vi "Moving_Avg_Filter.vi"(6 "Moving Array":dbl[][](array[numeric])) -> (3 "Output":dbl, 7 "Coefficients":dbl[](array[numeric]))   [LabVIEW 2016]
panel:
  out "size(s)":i32[](array[numeric])
  in  "Input":dbl[](array[numeric])
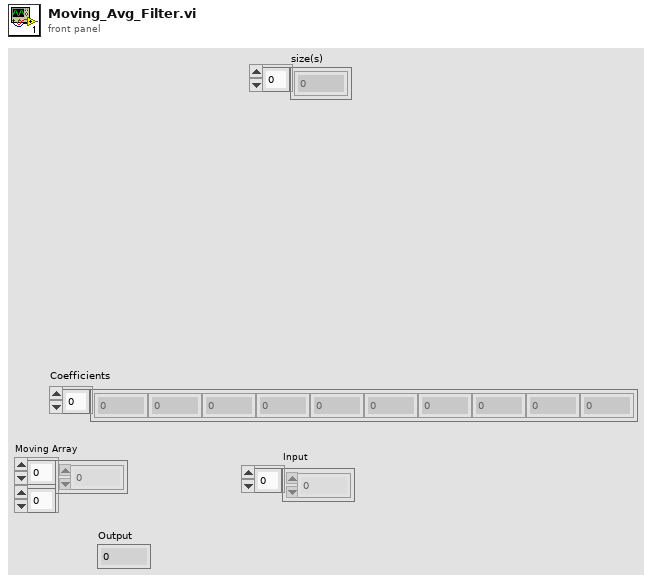
[diagram p1: front panel]
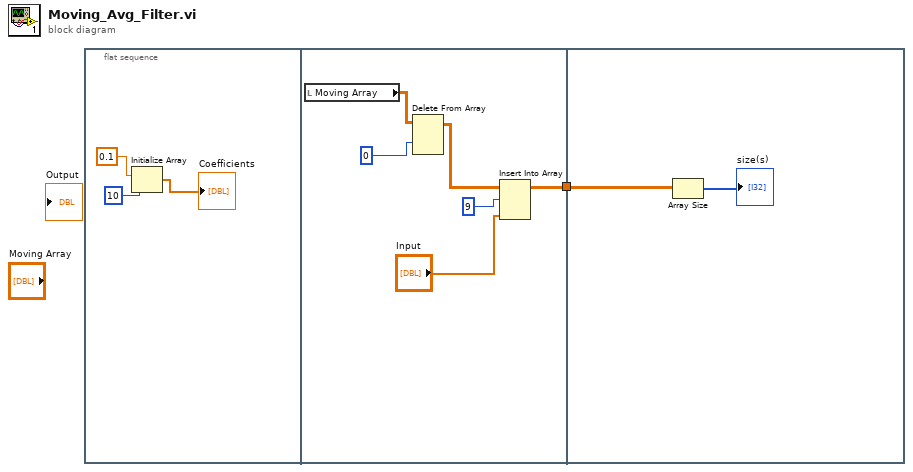
[diagram p0: block diagram]
diagram:
  n1 = flat-sequence {
    tunnel: [w5] -> w1
    tunnel: w1 -> [w12]
    frame #0 {
      n2 = Initialize Array(0.1 ("element"), 10 ("dimension size")) -> (→"Coefficients":dbl[])
    }
    frame #1 {
      n3 = local read "Moving Array"() -> (w10:dbl[][])
      n4 = Delete From Array(array=w10, index (row)=0) -> (array with subset deleted=w8:dbl[][])  [unwired: 2 in, 1 out]
      n5 = Insert Into Array(array=w8, index (row)=9, new element="Input") -> (w5:dbl[][])  [unwired: 1 in]
    }
    frame #2 {
      n6 = Array Size(array=w12) -> (size(s)=→"size(s)":i32[])
    }
  }
